vi "Read IMU Gyro.vi"(0 "I2CDevRef":T1={"DevStatus"={"status"=FALSE, "code"=0, "source"=""}, "Device Address"=0, "Handle"=0, "I2C Bus"=enum."Invalid"} {"Device Address" format="%.0x"}) -> (3 "I2CDevRef 2":T1={"DevStatus"={"status"=FALSE, "code"=0, "source"=""}, "Device Address"=0, "Handle"=0, "I2C Bus"=enum."Invalid"} {"Device Address" format="%.0x"}, 4 "X":dbl, 6 "Y":dbl, 8 "Z":dbl, 12 "Raw X":dbl, 13 "Raw Y":dbl, 14 "Raw Z":dbl)   [LabVIEW 2015]
uses:
  <vilib>/Rock Robotics/WPI/I2C/WPI_I2CDevRef.ctl
  <vilib>/Rock Robotics/SystemInterfaces/i2clib/i2c_bus.ctl
  Robot Global Data.vi
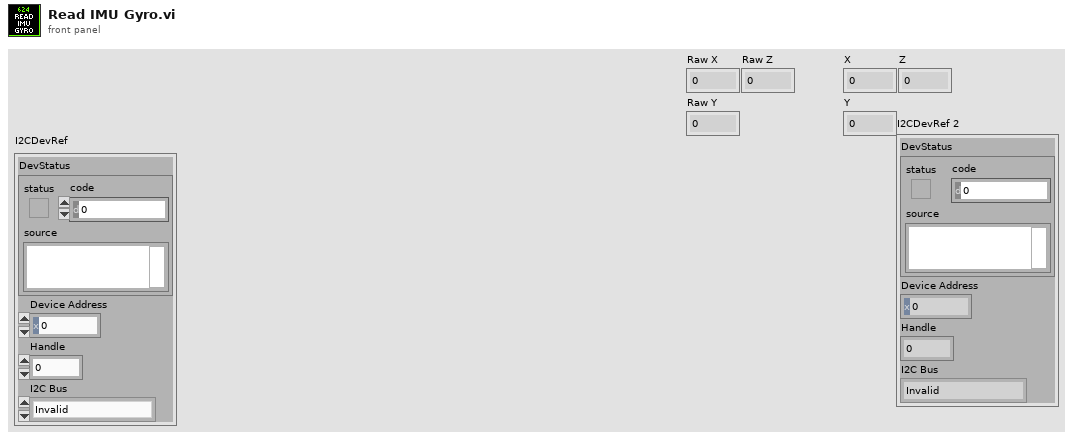
[diagram p1: front panel]
types:
  T1 = typedef "WPI_I2CDevRef.ctl" = cluster{"DevStatus":errorcluster, "Device Address":u8, "Handle":i32, "I2C Bus":T2}
  T2 = typedef "i2c_bus.ctl" = enum16{"I2C On-Board", "I2C MXP", "Invalid"}
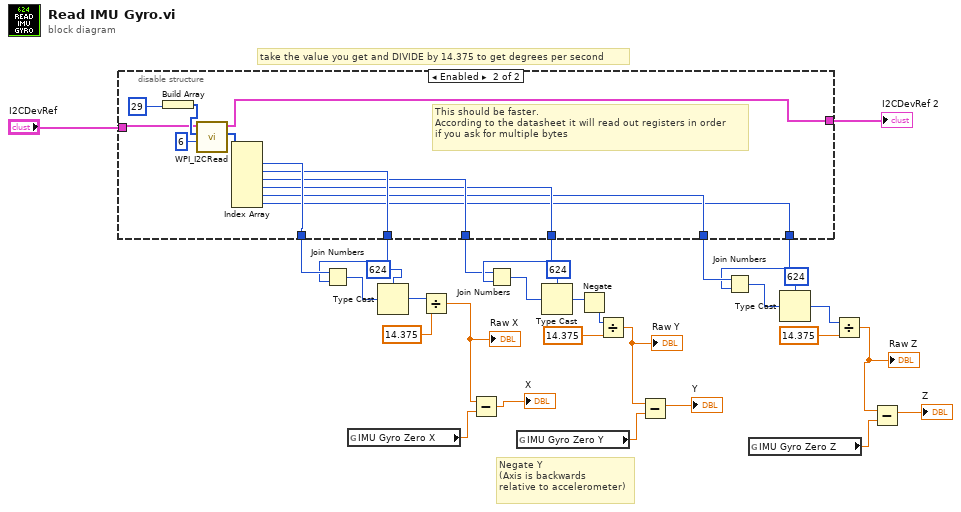
[diagram p0: block diagram]
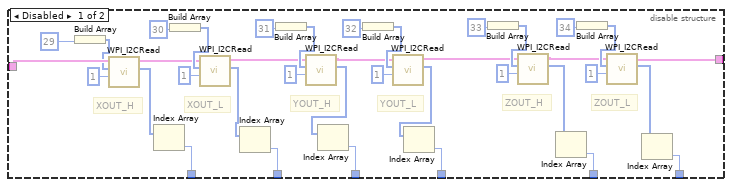
[diagram p2: hidden frame]
diagram:
  # "Negate Y\n(Axis is backwards\nrelative to accelerometer)"
  # "take the value you get and DIVIDE by 14.375 to get degrees per second"
  n1 = disable-structure shown="Enabled" {
    disable-tunnel: "I2CDevRef" -> [w67 w76]
    disable-tunnel: [w41 w74] -> w29
    disable-tunnel: [w40 w73] -> w28
    disable-tunnel: [w39 w71] -> w23
    disable-tunnel: [w38 w72] -> w22
    disable-tunnel: [w37 w70] -> w21
    disable-tunnel: [w36 w69] -> w20
    disable-tunnel: [w31 w68] -> w1
    frame Disabled {
      # "ZOUT_L"
      # "ZOUT_H"
      # "YOUT_L"
      # "YOUT_H"
      # "XOUT_L"
      # "XOUT_H"
      n2 = Build Array(u8 29) -> (w65:u8[])
      n3 = call <vilib>:"WPI_I2CRead.vi"("I2CBytesToRead"=u8 1, "I2CRegister"=w65, "I2CDevRef"=w67) -> ("Data Out"=w43:u8[], "I2CDevRef"=w60:T1)  [unwired: 6 in, 1 out]
      n4 = Index Array(array=w43) -> (element=w41:u8)  [unwired: 1 in]
      n5 = Build Array(u8 30) -> (w62:u8[])
      n6 = call <vilib>:"WPI_I2CRead.vi"("I2CBytesToRead"=u8 1, "I2CRegister"=w62, "I2CDevRef"=w60) -> ("Data Out"=w42:u8[], "I2CDevRef"=w56:T1)  [unwired: 6 in, 1 out]
      n7 = Index Array(array=w42) -> (element=w40:u8)  [unwired: 1 in]
      n8 = Build Array(u8 31) -> (w58:u8[])
      n9 = call <vilib>:"WPI_I2CRead.vi"("I2CBytesToRead"=u8 1, "I2CRegister"=w58, "I2CDevRef"=w56) -> ("Data Out"=w33:u8[], "I2CDevRef"=w52:T1)  [unwired: 6 in, 1 out]
      n10 = Index Array(array=w33) -> (element=w38:u8)  [unwired: 1 in]
      n11 = Build Array(u8 32) -> (w54:u8[])
      n12 = call <vilib>:"WPI_I2CRead.vi"("I2CBytesToRead"=u8 1, "I2CRegister"=w54, "I2CDevRef"=w52) -> ("Data Out"=w32:u8[], "I2CDevRef"=w44:T1)  [unwired: 6 in, 1 out]
      n13 = Index Array(array=w32) -> (element=w39:u8)  [unwired: 1 in]
      n14 = Build Array(u8 33) -> (w50:u8[])
      n15 = call <vilib>:"WPI_I2CRead.vi"("I2CBytesToRead"=u8 1, "I2CRegister"=w50, "I2CDevRef"=w44) -> ("Data Out"=w35:u8[], "I2CDevRef"=w45:T1)  [unwired: 6 in, 1 out]
      n16 = Index Array(array=w35) -> (element=w37:u8)  [unwired: 1 in]
      n17 = Build Array(u8 34) -> (w47:u8[])
      n18 = call <vilib>:"WPI_I2CRead.vi"("I2CBytesToRead"=u8 1, "I2CRegister"=w47, "I2CDevRef"=w45) -> ("Data Out"=w34:u8[], "I2CDevRef"=w31:T1)  [unwired: 6 in, 1 out]
      n19 = Index Array(array=w34) -> (element=w36:u8)  [unwired: 1 in]
    }
    frame Enabled {
      # "This should be faster.\nAccording to the datasheet it will read out registers in order\nif you ask for multiple bytes"
      n20 = Build Array(u8 29) -> (w78:u8[])
      n21 = call <vilib>:"WPI_I2CRead.vi"("I2CBytesToRead"=u8 6, "I2CRegister"=w78, "I2CDevRef"=w76) -> ("Data Out"=w75:u8[], "I2CDevRef"=w68:T1)  [unwired: 6 in, 1 out]
      n22 = Index Array(array=w75) -> (element #1=w74:u8, element #2=w73:u8, element #3=w72:u8, element #4=w71:u8, element #5=w70:u8, element #6=w69:u8)  [unwired: 6 in]
    }
  }
  "I2CDevRef 2" <- w1
  n23 = Join Numbers(hi=w29, lo=w28) -> ((hi.lo)=w27:u16)
  n24 = global read "Robot Global Data.vi" "IMU Gyro Zero X"() -> (w6:dbl)
  n25 = Type Cast(type=i16 624, x=w27) -> (*(type *) &x=w17:i16)
  n26 = Divide(x=w17, y=14.375) -> (x/y=w5:dbl)
  "Raw X" <- w5
  n27 = Subtract(x=w5, y=w6) -> (x-y=→"X":dbl)
  n28 = Join Numbers(hi=w22, lo=w23) -> ((hi.lo)=w24:u16)
  n29 = global read "Robot Global Data.vi" "IMU Gyro Zero Y"() -> (w9:dbl)
  n30 = Type Cast(type=i16 624, x=w24) -> (*(type *) &x=w3:i16)
  n31 = Negate(x=w3) -> (-x=w2:i16)
  n32 = Divide(x=w2, y=14.375) -> (x/y=w8:dbl)
  "Raw Y" <- w8
  n33 = Subtract(x=w8, y=w9) -> (x-y=→"Y":dbl)
  n34 = Join Numbers(hi=w21, lo=w20) -> ((hi.lo)=w19:u16)
  n35 = global read "Robot Global Data.vi" "IMU Gyro Zero Z"() -> (w11:dbl)
  n36 = Type Cast(type=i16 624, x=w19) -> (*(type *) &x=w13:i16)
  n37 = Divide(x=w13, y=14.375) -> (x/y=w12:dbl)
  "Raw Z" <- w12
  n38 = Subtract(x=w12, y=w11) -> (x-y=→"Z":dbl)
